vi "Update Filter.vi"(8 "error in":errorcluster, 11 "Refnum in":refnum<k21>) -> (0 "error out":errorcluster, 3 "Refnum out":refnum<k21>)   [LabVIEW 2015]
uses:
  Controls/Flags.ctl
  <vilib>/DAQmx/write.llb/DAQmx Write (Digital 1D Bool NChan 1Samp 1Line).vi
  <vilib>/DAQmx/miscellaneous.llb/DAQmx Fill In Error Info.vi
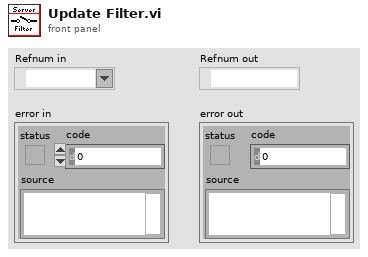
[diagram p1: front panel]
types:
  T1 = typedef "Flags.ctl" = enum8{"Autospeaker", "Link cycles", "Autofilter", "O3 Cal", "Filter Position"}
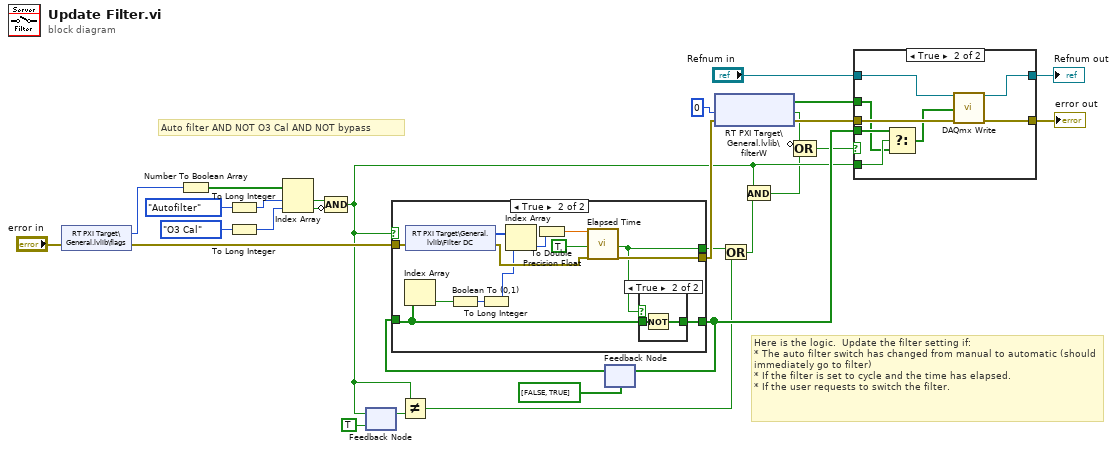
[diagram p0: block diagram]
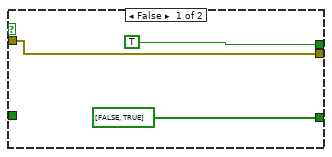
[diagram p2: hidden frame]
diagram:
  # "Auto filter AND NOT O3 Cal AND NOT bypass"
  # "Here is the logic.  Update the filter setting if:\n* The auto filter switch has changed from manual to automatic (should immediately go to filter)\n* If the filter is set to cycle and the time has elapsed.\n* If the user requests to switch the filter."
  n1 = shared-variable "RT PXI Target\\General.lvlib\\flags"(error in="error in") -> (w12:u8, error out=w19:errorcluster)
  n2 = Number To Boolean Array(number=w12) -> (Boolean array=w11:bool[])
  n3 = To Long Integer(number=Flags."Autofilter") -> (32bit integer=w1:i32)
  n4 = To Long Integer(number=Flags."O3 Cal") -> (32bit integer=w2:i32)
  n5 = Index Array(array=w11, index #1=w1, index #2=w2) -> (element #1=w10:bool, element #2=w9:bool)
  n6 = Compound Arithmetic op=AND(w10, invert w9) -> (w8:bool)
  n7 = feedback-in #1(w8) -> ()
  n8 = feedback #1(TRUE ("Boolean")) -> (w16:bool)
  n9 = Not Equal?(x=w8, y=w16) -> (x != y?=w15:bool)
  n10 = feedback #2(bool[] [FALSE, TRUE]) -> (w22:bool[])
  n11 = case shown="True" w8 {
    tunnel: [TRUE ("Time has Elapsed") w34] -> w17
    tunnel: [bool[] [FALSE, TRUE] w41] -> w20
    tunnel: w22 -> [_ w37]
    tunnel: w19 -> [w30 w40]
    tunnel: [w30 w38] -> w18
    frame False {
    }
    frame True {
      n12 = Index Array(array=w37) -> (element=w33:bool)  [unwired: 1 in]
      n13 = shared-variable "RT PXI Target\\General.lvlib\\Filter DC"(error in=w40) -> (w45:u16[], error out=w39:errorcluster)
      n14 = Boolean To (0,1)(Boolean=w33) -> (0, 1=w36:i16)
      n15 = To Long Integer(number=w36) -> (32bit integer=w35:i32)
      n16 = Index Array(array=w45, index=w35) -> (element=w44:u16)
      n17 = To Double Precision Float(number=w44) -> (double precision float=w43:dbl)
      n18 = call "Elapsed Time"("Time Target (s)"=w43, "Auto Reset"=TRUE, "error in (no error)"=w39) -> ("Time has Elapsed"=w34:bool, "error out"=w38:errorcluster)  [unwired: 9 in, 6 out]
      n19 = case shown="True" w34 {
        tunnel: w37 -> [w46 w48]
        tunnel: [w46 w47] -> w41
        frame False {
        }
        frame True {
          n20 = Not(x=w48) -> (.not. x?=w47:bool[])
        }
      }
    }
  }
  n21 = feedback-in #2(w20) -> ()
  n22 = shared-variable "RT PXI Target\\General.lvlib\\filterW"(error in=w18, 0 ("ms timeout (0)")) -> (w26:bool[], error out=w25:errorcluster, w5:bool)
  n23 = Or(x=w17, y=w15) -> (x .or. y?=w14:bool)
  n24 = And(x=w8, y=w14) -> (x .and. y?=w7:bool)
  n25 = Compound Arithmetic op=OR(invert w5, w7) -> (w6:bool)
  n26 = case shown="True" w6 {
    tunnel: w25 -> [w49 w58]
    tunnel: [w49 w57] -> w29
    tunnel: [w50 w56] -> w28
    tunnel: "Refnum in" -> [w50 w55]
    tunnel: w26 -> [_ w52]
    tunnel: w8 -> [_ w54]
    tunnel: w20 -> [_ w53]
    frame False {
    }
    frame True {
      n27 = Select(t=w53, s=w54, f=w52) -> (s? t:f=w51:bool[])
      n28 = call-poly <vilib>:"DAQmx Write.vi"("task/channels in"=w55, "data"=w51, "error in"=w58) -> ("task out"=w56:refnum<k21>, "error out"=w57:errorcluster)  [unwired: 10 in, 1 out]
    }
  }
  "error out" <- w29
  "Refnum out" <- w28
